vi "Simple Lossy Class.vi"() -> ()   [LabVIEW 2022 SP3]
uses:
  Enclave/Enclave.lvlib
  Enclave/Tag/Tag.lvclass
  Enclave/Writer/Writer.lvclass
  Enclave/Lossless/Lossless.lvclass
  Enclave/Element.ctl
panel:
  out "Chart 2":dbl(graph)
  out "Chart":dbl(graph)
  in  "stop 3":bool
  in  "stop 2":bool
  out "Sequence 2":u64
  out "Time Stamp 2":timestamp
  out "Element 3":T1
  in  "stop":bool
  in  "Element":T1
  out "Element 2":T1
  out "Time Stamp":timestamp
  out "Sequence":u64
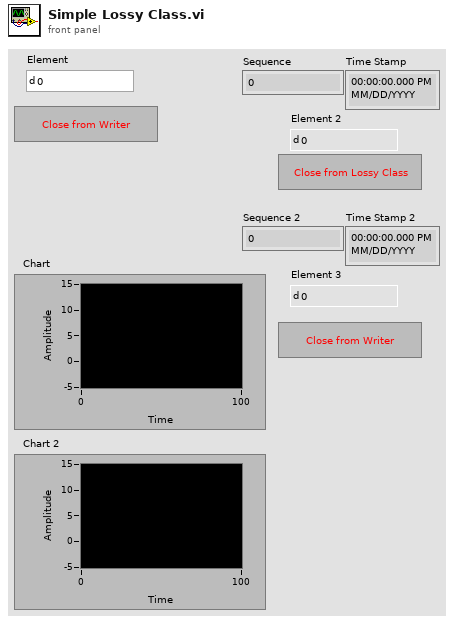
[diagram p1: front panel]
types:
  T1 = typedef "Enclave.lvlib/Element.ctl" = dbl
  T2 = typedef "Enclave.lvlib/))Channel.ctl" = refnum<queue>
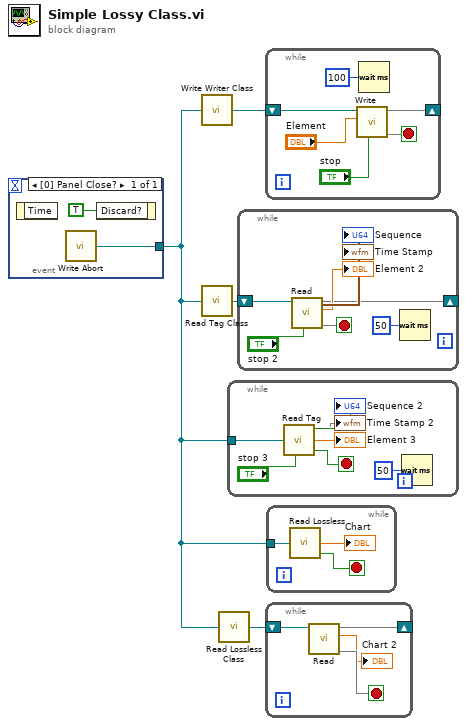
[diagram p0: block diagram]
diagram:
  n1 = call "Read Tag Class.vi"() -> ("EnclaveChannel"=w1:T2, "Lossy Reader"=w4:refnum<class "Tag.lvclass">)  [unwired: 7 in, 1 out]
  n2 = event shown="[0] Panel Close?" {
    selector: _ -> [_]
    dyn-events: _ -> [_]
    timeout: _ -> [_]
    tunnel: w1 -> [w5]
    event Panel Close? {
      n3 = event-data() -> ()  [unwired: 1 in, 1 out]
      n4 = call "Write Abort.vi"("EnclaveChannel"=w5) -> ()
      n5 = event-data("Discard?"=TRUE) -> ()  [unwired: 1 in, 1 out]
    }
  }
  n6 = call "Write Writer Class.vi"("EnclaveChannel"=w1) -> ("Writer"=w3:refnum<class "Writer.lvclass">)  [unwired: 8 in]
  n7 = call "Read Lossless Class.vi"("EnclaveChannel"=w1) -> ("Lossless"=w2:refnum<class "Lossless.lvclass">)  [unwired: 7 in, 1 out]
  n8 = while {
    tunnel: w1 -> [w12]
    stop <- w8 stop-if-true
    n9 = call "Read Tag.vi"("EnclaveChannel"=w12, 4:"stop 3") -> ("New Value?"=→"Sequence 2":bool, 6:→"Time Stamp 2", "Element"=→"Element 3":T1, "timed out?"=w8:bool)  [unwired: 2 in, 2 out]
    n10 = Wait (ms)(milliseconds to wait=u32 50) -> ()  [unwired: 1 out]
  }
  n11 = while {
    shift-right: [w16] -> _
    shift-left: w4 -> [w21]
    stop <- w15 stop-if-true
    n12 = call "Read.vi"(6:"stop 2", "Tag in"=w21) -> (0:w15, "Element"=→"Element 2":T1, 3:w16, "New Value?"=→"Time Stamp":bool, "Time Stamp"=→"Sequence":timestamp)  [unwired: 3 in, 2 out]
    n13 = Wait (ms)(milliseconds to wait=u32 50) -> ()  [unwired: 1 out]
  }
  n14 = while {
    shift-right: [w25] -> _
    shift-left: w3 -> [w27]
    stop <- w23 stop-if-true
    n15 = call "Write.vi"("Close (F)"="stop", "Element"="Element", "Writer in"=w27) -> (0:w23, 3:w25)  [unwired: 5 in, 2 out]
    n16 = Wait (ms)(milliseconds to wait=u32 100) -> ()  [unwired: 1 out]
  }
  n17 = while {
    shift-right: [w28] -> _
    shift-left: w2 -> [w31]
    stop <- w30 stop-if-true
    n18 = call "Read.vi"("Lossless in"=w31) -> (0:w30, "Element"=→"Chart 2":T1, 3:w28)  [unwired: 6 in, 2 out]
  }
  n19 = while {
    tunnel: w1 -> [w34]
    stop <- w33 stop-if-true
    n20 = call "Read Lossless.vi"("EnclaveChannel"=w34) -> ("Element"=→"Chart":T1, "timed out?"=w33:bool)  [unwired: 6 in, 1 out]
  }
